vi "Remove Map of Created Attributes.vi"(10 "Alias":string, 11 "Base Actor in":refnum<class "Base Actor.lvclass">) -> (3 "Base Actor out":refnum<class "Base Actor.lvclass">)   [LabVIEW 2020, in "jettl.lvlib" / "Actor.lvlib" / "Base Actor.lvclass"]
uses:
  Base Actor.lvclass
  Base Actor.lvclass/Base Actor.ctl
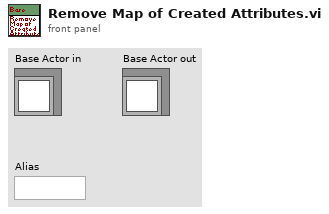
[diagram p1: front panel]
types:
  T1 = typedef "jettl.lvlib/Actor.lvlib/Map of Created Attributes.ctl" = map{string, refnum<class "Attributes.lvclass">}
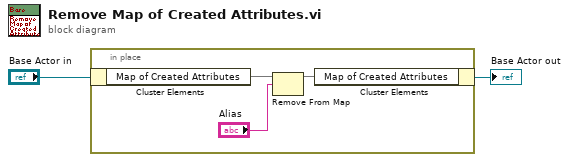
[diagram p0: block diagram]
diagram:
  n1 = in-place {
    n2 = in-place-cluster #1("Base Actor in") -> ("Map of Created Attributes"=w5:T1)
    n3 = Remove From Map(10:"Alias", 11:w5) -> (3:w4:T1)  [unwired: 2 out]
    n4 = in-place-cluster #1("Map of Created Attributes"=w4) -> (→"Base Actor out":refnum<class "Base Actor.lvclass">)
  }
